vi "Take multiple measurements.vi"() -> ()   [LabVIEW 2017, in "GP22_TDC_Arduinoed.lvlib"]
uses:
  GP22_TDC_Arduinoed.lvlib
panel:
  in  "# bins":i32=100
  in  "Time in ms (30000)":u32=5000
  out "Timing histogram":T1(graph)
  out "error out":errorcluster
  in  "VISA resource name":refnum<visa-resource-name>
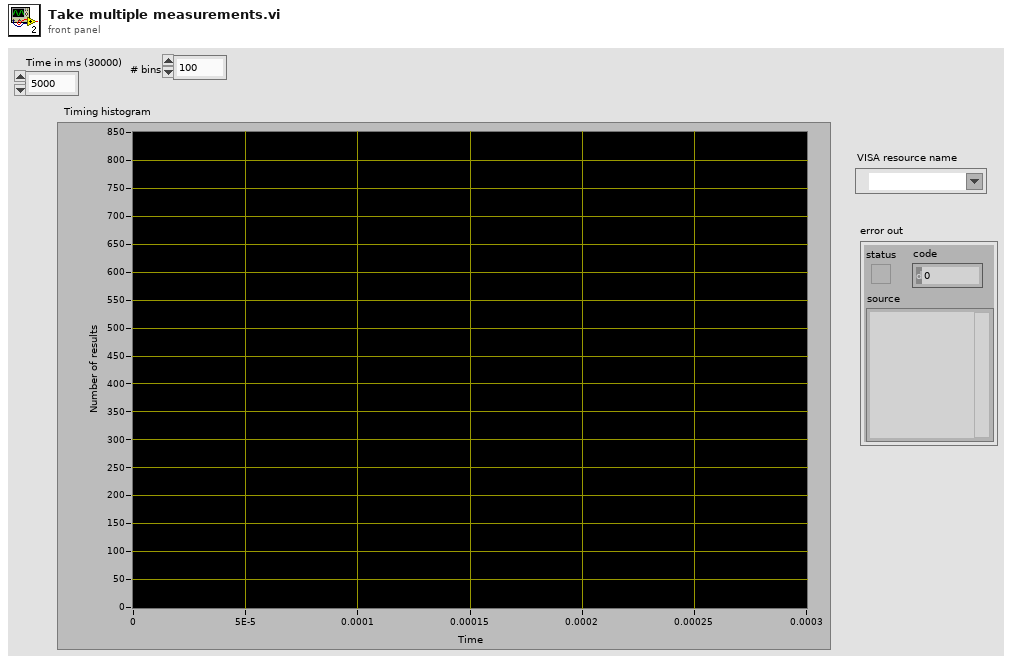
[diagram p1: front panel]
types:
  T1 = cluster{"Unbinned times / s":dbl[], "Binned time":dbl[]}
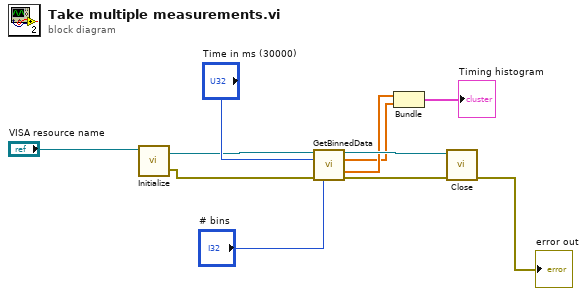
[diagram p0: block diagram]
diagram:
  n1 = call "Initialize.vi"("VISA resource name"="VISA resource name") -> ("error out"=w7:errorcluster, "VISA resource name out"=w9:refnum<visa-resource-name>)  [unwired: 5 in]
  n2 = call "GetBinnedData.vi"("VISA resource name"=w9, "Time in ms (30000)"="Time in ms (30000)", "error in"=w7, "# bins"="# bins") -> ("VISA resource name out"=w8:refnum<visa-resource-name>, "Binned time"=w3:dbl[], "Unbinned times / s"=w4:dbl[], "error out"=w6:errorcluster)  [unwired: 8 in]
  n3 = Bundle("Unbinned times / s"=w4, "Binned time"=w3) -> (→"Timing histogram":T1)  [unwired: 1 in]
  n4 = call "Close.vi"("error in (no error)"=w6, "VISA resource name"=w8) -> ("error out"=→"error out":errorcluster)  [unwired: 9 in]
